vi "Dashboard Main.vi"() -> ()   [LabVIEW 2015]
uses:
  <vilib>/Utility/miscctls.llb/LVRowAndColumnTypeDef.ctl
  <vilib>/event_ctls.llb/eventvkey.ctl
  <vilib>/Rock Robotics/WPI/Dashboard/WPI_DashboardLogging Global.vi
  <vilib>/Rock Robotics/Network Tables/NT Read Boolean.vi
  <vilib>/Rock Robotics/Network Tables/NT Read Numeric Array.vi
  <vilib>/Utility/config.llb/Write Key (String).vi
  <vilib>/Utility/config.llb/Write Key (I32).vi
  <vilib>/Utility/config.llb/NI_LVConfig.lvlib
  <vilib>/vision/NI_Vision_Development_Module.lvlib
panel:
  out "Camera Image 2":T1(plugin-control)
  in  "Vision 2":u16(ring) items=["Camera Off", "USB Camera SW", "USB Camera HW", "IP Camera"]
  in  "Rec Mode":enum32{"Stop", "Record", "Playback"}(radio)
  in  "Vision":u16(ring) items=["Camera Off", "USB Camera SW", "USB Camera HW", "IP Camera"]
  in  "Dashboard Tab":T2(tab)
  out "Camera Reversed":bool
  out "dist":dbl
  in  "Select Auto":string(combo)
  out "NT Connection":bool
  in  "Camera Settings":T3={"Frame Rate"=30, "Compression"=30, "Size"=1} {"Frame Rate" scale=1.0..30.0; "Size" items=["640x480", "320x240", "160x120"]}
  out "MotorChart R":cluster{"Numeric":dbl, "Numeric":dbl}(graph)
  out "MotorChart L":T4(graph)
  out "MotorSliders R":cluster{"MotorSlide1":dbl, "MotorSlide2":dbl} {"MotorSlide2" scale=-1.0..1.0 scale format="%#_2e"; "MotorSlide1" scale=-1.0..1.0 scale format="%#_2e"}
  out "MotorSliders L":T5 {"MotorSlide4 2" scale=0.0..14.0 scale format="%#_2e"; "MotorSlide2" scale=-1.0..1.0 scale format="%#_2e"; "MotorSlide1" scale=-1.0..1.0 scale format="%#_2e"}
  out "Gyro":dbl(knob) scale=0.0..360.0
  out "JS1 Z":dbl(slide) scale=-1.0..1.0 scale format="%#_2e"
  out "JS1 Graph":cluster{"X":dbl, "Y":dbl}[](graph)
  out "JS1 Buttons":T6
  out "JS2 Z":dbl(slide) scale=-1.0..1.0 scale format="%#_2e"
  out "JS2 Graph":cluster{"X":dbl, "Y":dbl}[](graph)
  out "JS2 Buttons":T6
  out "Mode":T7(ring)=enum."Auto Disabled"
  in  "DB Camera Config":bool
  out "fps":dbl format="%#.1g"
  out "Mbps":dbl format="%#.1g"
  out "Mbps LED":bool
  in  "Camera Settings 2":T3={"Frame Rate"=30, "Compression"=30, "Size"=1} {"Frame Rate" scale=1.0..30.0; "Size" items=["640x480", "320x240", "160x120"]}
  out "Mbps 2":dbl format="%#.1g"
  out "fps 2":dbl format="%#.1g"
  out "Background":bool
  in  "DB/String 9":string
  in  "DB/String 8":string
  in  "DB/String 7":string
  in  "DB/String 6":string
  in  "DB/String 5":string
  in  "DB/String 4":string
  in  "DB/String 3":string
  in  "DB/String 2":string
  in  "DB/String 1":string
  in  "DB/String 0":string
  in  "DB/Slider 0":dbl(slide) scale=0.0..5.0
  in  "DB/Slider 1":dbl(slide) scale=0.0..5.0
  in  "DB/Slider 2":dbl(slide) scale=0.0..5.0
  in  "DB/Slider 3":dbl(slide) scale=0.0..5.0
  out "DB/LED 3":bool
  out "DB/LED 2":bool
  out "DB/LED 1":bool
  out "DB/LED 0":bool
  in  "DB/Button 3":bool
  in  "DB/Button 2":bool
  in  "DB/Button 1":bool
  in  "DB/Button 0":bool caption="New Name"
  in  "Test Slider":dbl(slide) scale=0.0..100.0 scale format="%#_3g"
  in  "On/Off":bool caption="Solenoid"
  in  "Test Name":u16(ring) items=["Select the test to run..."]
  in  "Test Tree":string(tree)
  in  "Motor":cluster{"Value":dbl, "Enable":bool} {"Value" scale=-1.0..1.0 scale format="%#_3g"}
  out "Progress":T8 {"Test Progress" scale=0.0..100.0}
  in  "Rev/Fwd":cluster{"Forward":bool, "Reverse":bool}
  in  "Test Ring":u16(ring) items=["Monochrome", "Color"]
  out "Cmd Status":string
  in  "Execute Command":bool
  in  "Command Params":string[][](table)
  in  "Command Selection":i32(listbox)
  in  "CheckList":i32(listbox)
  out "Tree":string(tree)
  in  "TCP":refnum<k5>
  out "Camera IP":string
  out "Image Message":string="Timeout in Camera Communications"
  out "Camera Image":T1(plugin-control)
  # "Left"
  # "Front"
  # "Right"
  # "Battery"
  # "This tab is a great place for autonomous settings and robot-specific values.\nPlace controls and indicators inside this tab and match name to\nDashboard Variables on robot. You can also delete this comment."
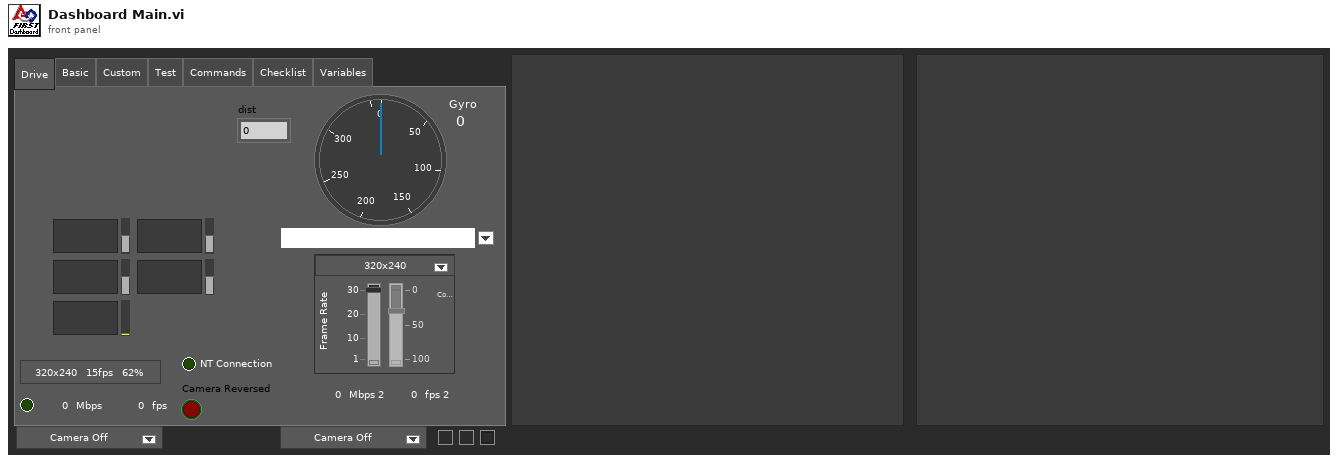
[diagram p1: front panel]
types:
  T1 = typedef "IMAQ Image.ctl" = refnum<image>
  T2 = enum32{"Drive", "Basic", "Custom", "Test", "Commands", "Checklist", "Variables"}
  T3 = cluster{"Frame Rate":i32, "Compression":i32, "Size":u16}
  T4 = cluster{"Numeric":dbl, "Numeric":dbl, "Battery V":dbl}
  T5 = cluster{"MotorSlide1":dbl, "MotorSlide2":dbl, "MotorSlide4 2":dbl}
  T6 = cluster{bool, bool, bool, bool, bool, bool, bool, bool, bool, bool, bool, bool}
  T7 = enum8{"Tele-Op Disabled", "Tele-Op Enabled", "Auto Disabled", "Auto Enabled", "Test Disabled", "Test Enabled", "Disconnected", "No Code", "E-Stop"}
  T8 = cluster{"Test Progress":u8, "Test Progress Text":string}
  T9 = typedef "Image Type" = u32
  T10 = cluster{"IDs":cluster{"RPC field ID":u16, "Unique ID":u16}, "String":string}
  T11 = enum32{"Drive", "Basic", "Custom", "Test", "Checklist", "Variables"}
  T12 = cluster{"Camera Image":refnum<vi>, "Dashboard Tab":refnum<vi>, "Background":refnum<vi>, "Vision":refnum<vi>, "Rec Mode":refnum<vi>, "Test Slider":refnum<vi>, "On/Off ":refnum<vi>, "Test Ring":refnum<vi>, "Rev/Fwd":refnum<vi>, "Test Name":refnum<vi>, "Motor":refnum<vi>, "Progress":refnum<vi>, "CheckList":refnum<vi>, "Tree":refnum<vi>, "Test Tree":refnum<vi>, "Command Params":refnum<vi>, "Command Selection":refnum<vi>, "Execute Command":refnum<vi>, "Cmd Status":refnum<vi>}
  T13 = cluster{"Error Strings":string, "Disable Counts":cluster{u16, u16}, "Rail Faults":cluster{u16, u16, u16}, "Robot IP":string, "DB Mode":u8, "Event Info":cluster{"Name":string, "Type":u8, "Number":u16, "Replay":u8}, "Camera Addr":string}
  T14 = cluster{"Storage":cluster{"Disk Free":u64, "RAM Block":u32, "RAM free":u32}, "CPU Utilization":cluster{"CPU % ISR":sgl, "CPU % Time Crit":sgl, "CPU % Timed Str":sgl, "CPU % High":sgl, "CPU % Above":sgl, "CPU % Normal":sgl, "CPU % Low":sgl}, "CAN":cluster{"% Bus Utilization":sgl, "Bus Off Cnt":u32, "TX_FIFO Full Cnt":u32, "Receive Error Cnt":u8, "Transmit Error Cnt":u8}, "HID":cluster{"HID Outputs":u32, "Rumble Low":u16, "Rumble High":u16}[]}
  T15 = cluster{"Status bits":cluster{"Test Mode":bool, "Autonomous":bool, "Enabled":bool, "Code Start":bool, "Brownout":bool, "Reserved 2":bool, "Reserved 3":bool, "E-Stop":bool}, "Code Trace":cluster{"Disabled":bool, "TeleOp":bool, "Auto":bool, "Test":bool}, "Controller Type":enum16{"unknown", "cRIO", "roboRio"}, "Code?":enum16{"unknown", "noCode", "code"}, "Battery V":dbl}
  T16 = cluster{"Control Bits":cluster{"TestMode":bool, "Autonomous":bool, "Enabled":bool, "FMS Present":bool, bool, bool, bool, "E-Stop":bool}, "Team Station ":u8, "Countdown":sgl, "Joystick Values":cluster{"Axes":dbl[], "Buttons":bool[], "POVs":i16[]}[]}
  T17 = cluster{"Axes":dbl[], "Buttons":bool[], "POVs":i16[]}[]
  T18 = cluster{"Axes":dbl[], "Buttons":bool[], "POVs":i16[]}
  T19 = cluster{"Buttons[0]":bool, "Buttons[1]":bool, "Buttons[2]":bool, "Buttons[3]":bool, "Buttons[4]":bool, "Buttons[5]":bool, "Buttons[6]":bool, "Buttons[7]":bool, "Buttons[8]":bool, "Buttons[9]":bool, "Buttons[10]":bool, "Buttons[11]":bool}
  T20 = typedef "NI_LVConfig.lvlib/Config Data RefNum.ctl" = refnum<k1>
  T21 = cluster{"Operation":enum16{"Update", "Clear"}, "Color Box":u32}[]
  T22 = typedef "eventvkey.ctl" = enum16{"ASCII", "Enter", "Return", "Shift", "Ctrl", "Alt", "Cmd", "Opt", "Caps", "NumLock", "Clear", "Break", "Up", "Down", "Left", "Right", "Insert", "Delete", "Home", "End", "PageUp", "PageDown", "Escape", "Help", "Pause", "ScrollLock", "F1", "F2", "F3", "F4", "F5", "F6", "F7", "F8", "F9", "F10", "F11", "F12", "F13", "F14", "F15", "F16", "F17", "F18", "F19", "F20", "F21", "F22", "F23", "F24", "Play", "VolumeUp", "VolumeDown", "Mute", "Two Byte Char"}
  T23 = cluster{"Image Size":bool, "Image Type":bool, "Pixel Value":bool, "ROI Information":bool, "Zoom Factor":bool}
  T24 = enum8{"Enabled", "Disabled", "Disabled and Grayed Out"}
  T25 = cluster{"Operation":enum16{"Update", "Clear"}, "Color Box":u32}
  T26 = typedef "LVRowAndColumnTypeDef.ctl" = cluster{"Row":i32, "Column":i32}
  T27 = cluster{"Shift":bool, "Ctrl":bool, "Alt":bool, "Cmd":bool, "Opt":bool}
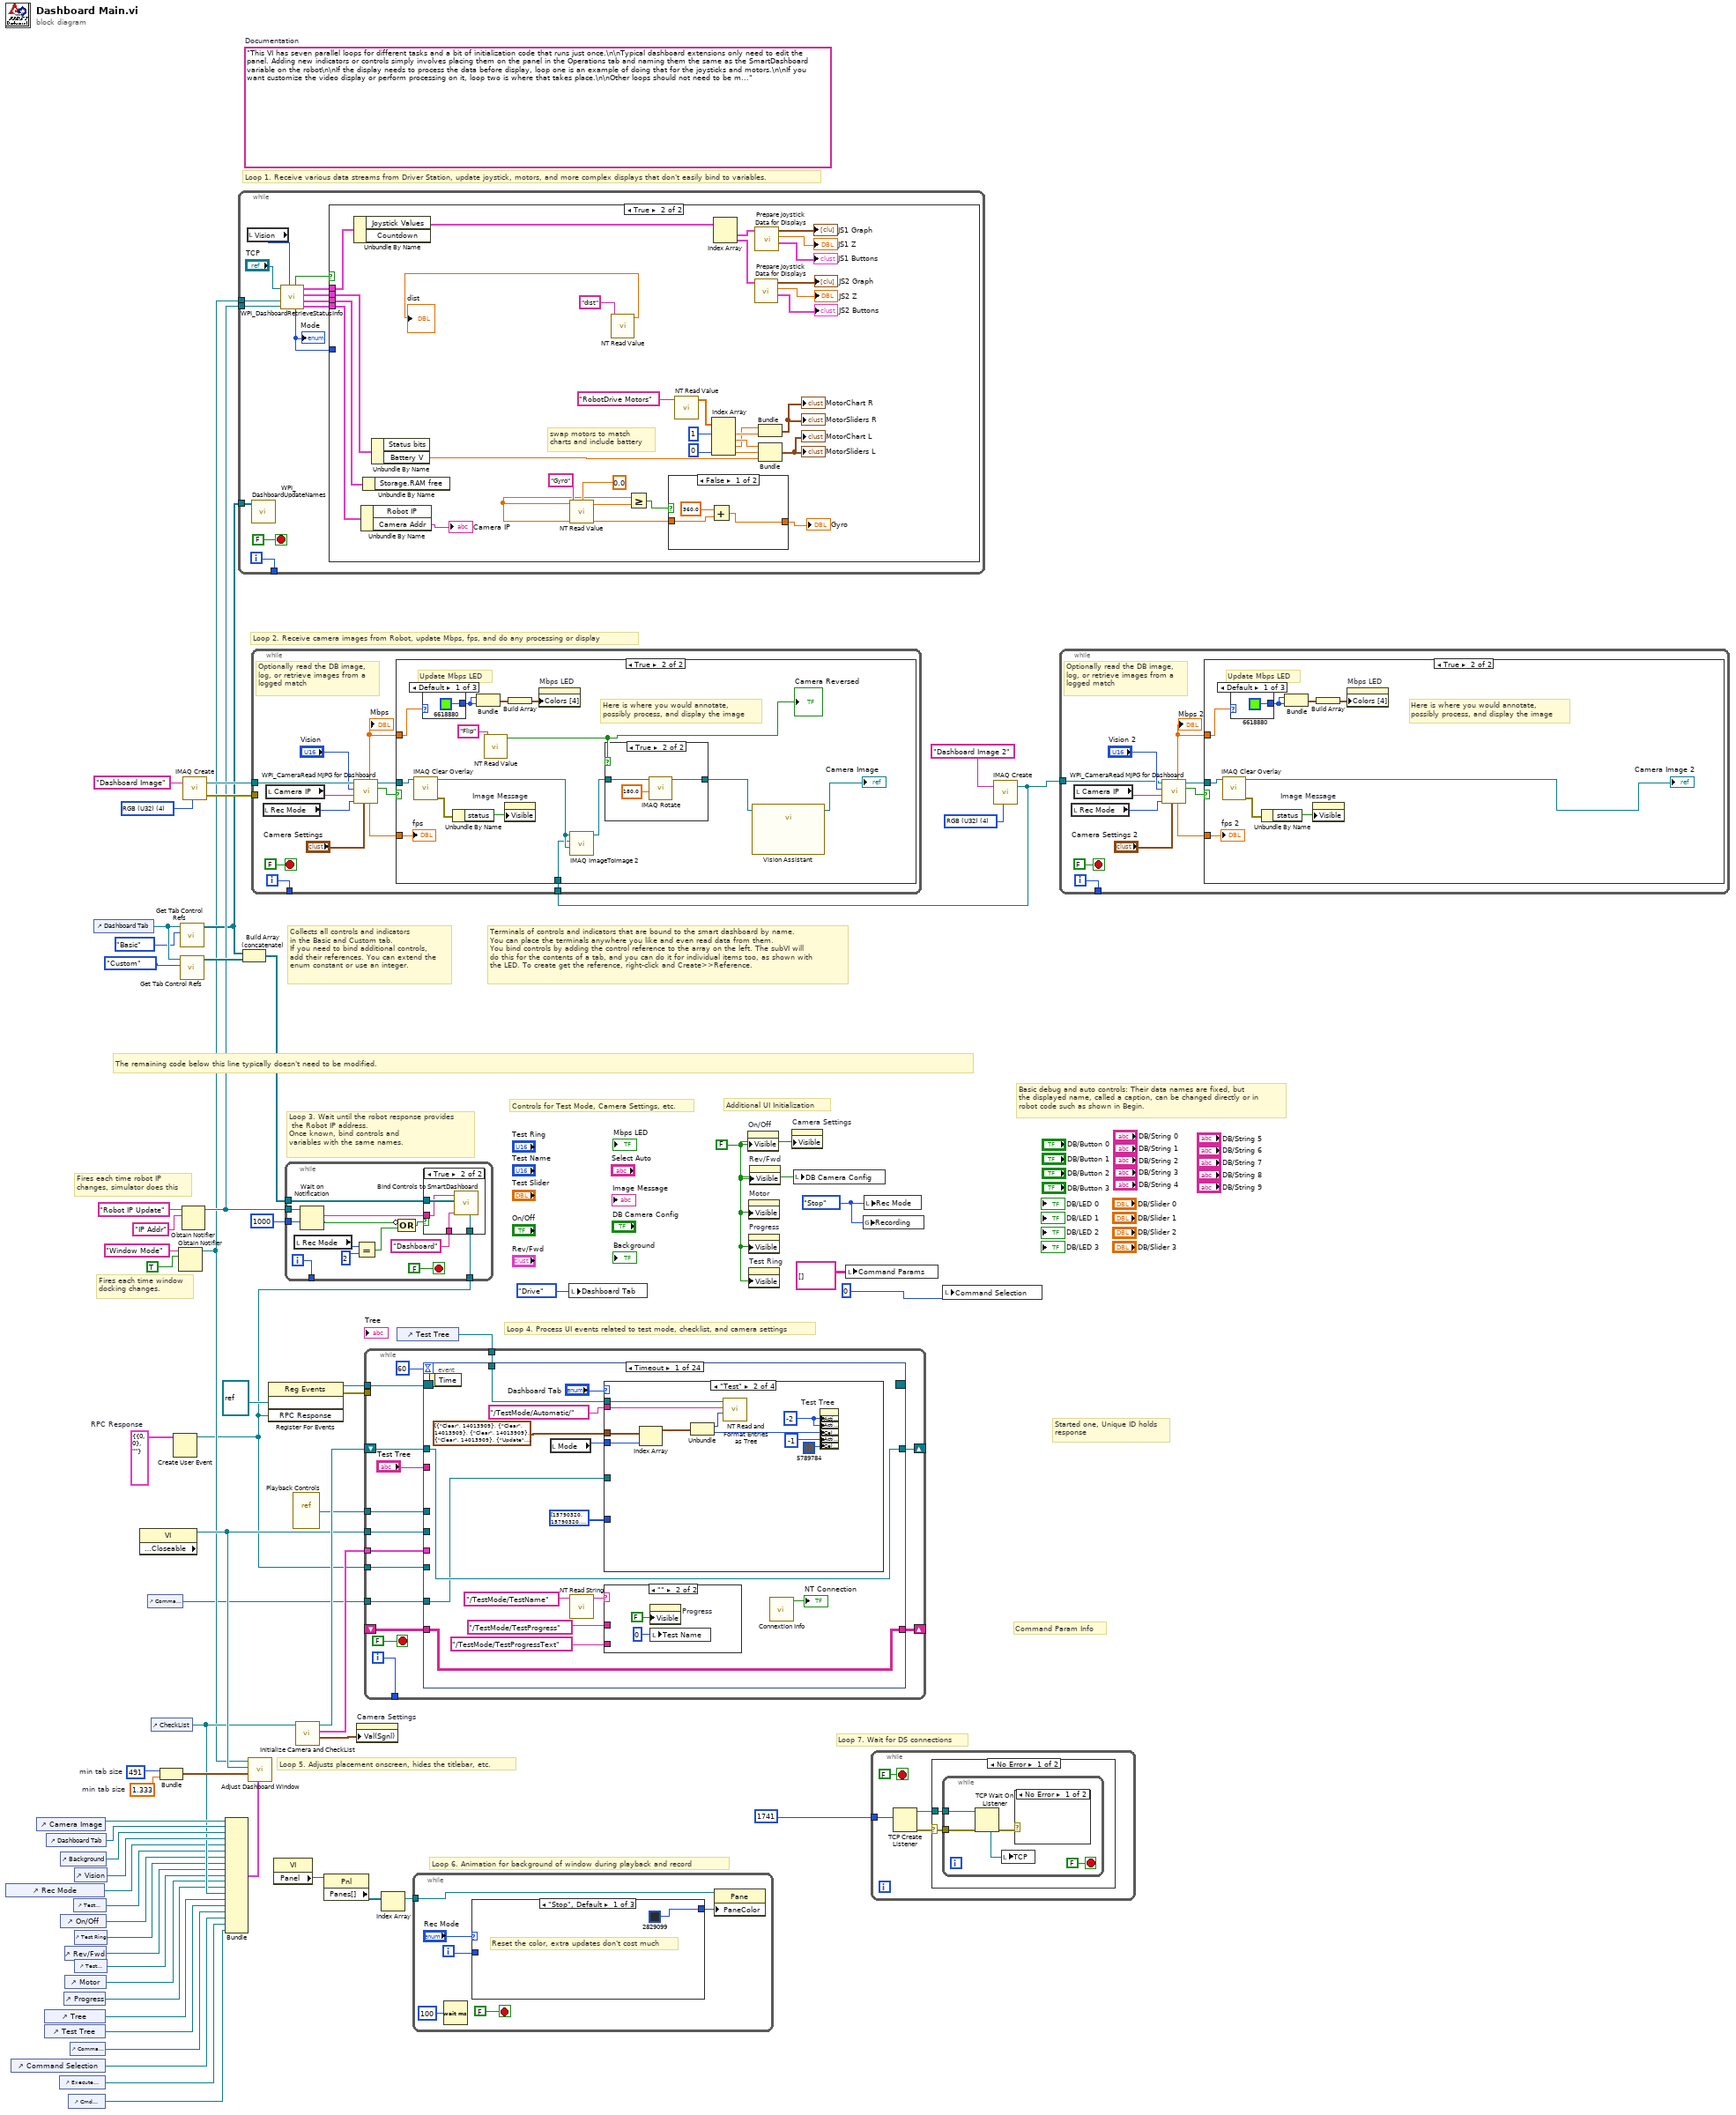
[diagram p0: block diagram]
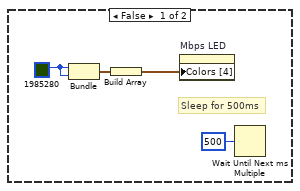
[diagram p2: hidden frame]
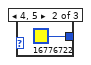
[diagram p3: hidden frame]
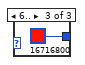
[diagram p4: hidden frame]
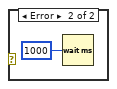
[diagram p5: hidden frame]
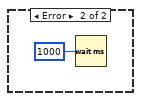
[diagram p6: hidden frame]
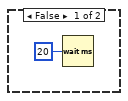
[diagram p7: hidden frame]
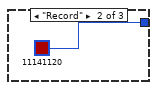
[diagram p9: hidden frame]
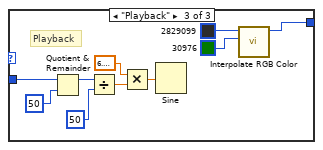
[diagram p10: hidden frame]
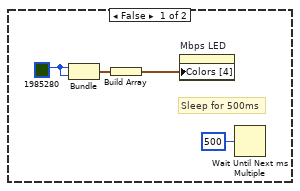
[diagram p12: hidden frame]
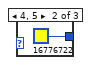
[diagram p14: hidden frame]
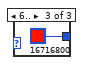
[diagram p15: hidden frame]
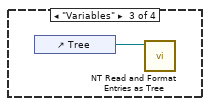
[diagram p17: hidden frame]
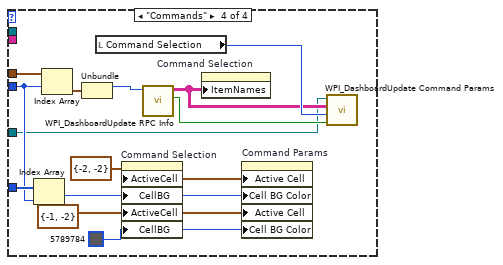
[diagram p18: hidden frame]
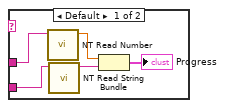
[diagram p19: hidden frame]
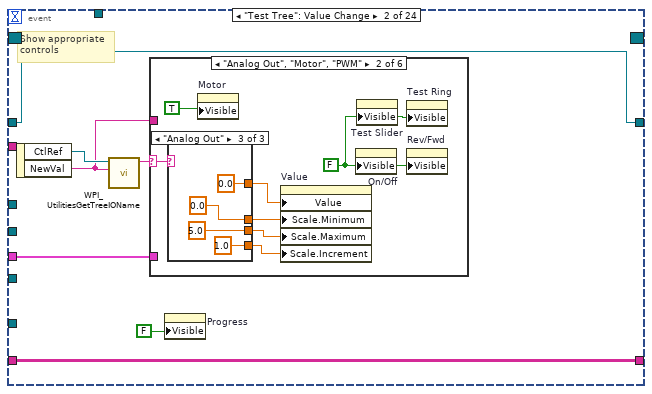
[diagram p20: hidden frame]
diagram:
  w2 = T9 4 items=["Grayscale (U8)", "Grayscale (I16)", "Grayscale (SGL)", "Complex (CSG)", "RGB (U32)", "HSL (U32)", "RGB (U64)", "Grayscale (U16)"] ("Image Type")
  w10 = T10 {"IDs"={"RPC field ID"=0, "Unique ID"=0}, "String"=""}  # RPC Response
  w36 = 491  # min tab size
  w35 = 1.333  # min tab size
  w44 = enum32{"Stop", "Record", "Playback"}."Stop" ("Rec Mode")
  w18 = FALSE ("Visible")
  (unwired) "This VI has seven parallel loops for different tasks and a bit of initialization code that runs just once.\n\nTypical dashboard extensions only need to edit the panel. Adding new indicators or controls simply involves placing them on the panel in the Operations tab and naming them the same as the SmartDashboard variable on the robot\n\nIf the display needs to process the data before display, loop one is an example of doing that for the joysticks and motors.\n\nIf you want customize the video display or perform processing on it, loop two is where that takes place.\n\nOther loops should not need to be modified. They are pretty standard, and document the task they perform."  # Documentation
  w64 = T9 4 items=["Grayscale (U8)", "Grayscale (I16)", "Grayscale (SGL)", "Complex (CSG)", "RGB (U32)", "HSL (U32)", "RGB (U64)"] ("Image Type")
  # "Command Param Info"
  # "Started one, Unique ID holds\nresponse"
  # "Loop 7. Wait for DS connections"
  # "Basic debug and auto controls: Their data names are fixed, but\nthe displayed name, called a caption, can be changed directly or in\nrobot code such as shown in Begin."
  # "Controls for Test Mode, Camera Settings, etc."
  # "Additional UI Initialization"
  # "Loop 6. Animation for background of window during playback and record"
  # "Fires each time robot IP\nchanges, simulator does this"
  # "Fires each time window\ndocking changes."
  # "Collects all controls and indicators\nin the Basic and Custom tab.\nIf you need to bind additional controls,\nadd their references. You can extend the\nenum constant or use an integer."
  # "The remaining code below this line typically doesn't need to be modified."
  # "Loop 4. Process UI events related to test mode, checklist, and camera settings"
  # "Terminals of controls and indicators that are bound to the smart dashboard by name.\nYou can place the terminals anywhere you like and even read data from them.\nYou bind controls by adding the control reference to the array on the left. The subVI will\ndo this for the contents of a tab, and you can do it for individual items too, as shown with\nthe LED. To create get the reference, right-click and Create>>Reference."
  # "Loop 3. Wait until the robot response provides\n the Robot IP address.\nOnce known, bind controls and\nvariables with the same names."
  # "Loop 5. Adjusts placement onscreen, hides the titlebar, etc."
  # "Loop 1. Receive various data streams from Driver Station, update joystick, motors, and more complex displays that don't easily bind to variables."
  # "Loop 2. Receive camera images from Robot, update Mbps, fps, and do any processing or display"
  n1 = control-ref of="Rec Mode"() -> (w24:refnum<vi>)
  n2 = control-ref of="Command Selection"() -> (w9:refnum<vi>)
  n3 = control-ref of="Camera Image"() -> (w39:refnum<vi>)
  n4 = control-ref of="Tree"() -> (w28:refnum<vi>)
  n5 = control-ref of="Test Tree"() -> (w27:refnum<vi>)
  n6 = control-ref of="Dashboard Tab"() -> (w38:refnum<vi>)
  n7 = control-ref of="Execute Command"() -> (w11:refnum<vi>)
  n8 = control-ref of="Background"() -> (w33:refnum<vi>)
  n9 = control-ref of="On/Off"() -> (w22:refnum<vi>)
  n10 = control-ref of="Progress"() -> (w19:refnum<vi>)
  n11 = control-ref of="Rev/Fwd"() -> (w20:refnum<vi>)
  n12 = control-ref of="Motor"() -> (w25:refnum<vi>)
  n13 = control-ref of="Cmd Status"() -> (w5:refnum<vi>)
  n14 = control-ref of="Command Params"() -> (w12:refnum<vi>)
  n15 = control-ref of="Test Slider"() -> (w23:refnum<vi>)
  n16 = control-ref of="Vision"() -> (w37:refnum<vi>)
  n17 = control-ref of="Test Ring"() -> (w21:refnum<vi>)
  n18 = control-ref of="Test Name"() -> (w26:refnum<vi>)
  n19 = control-ref of="Dashboard Tab"() -> (w42:refnum<vi>)
  n20 = property class="VI" props=["Front Panel.Closeable"]() -> (reference out=w43:refnum<vi>)  [unwired: 2 in, 2 out]
  n21 = control-ref of="Command Params"() -> (w4:refnum<vi>)
  n22 = control-ref of="CheckList"() -> (w29:refnum<vi>)
  n23 = Bundle("min tab size"=w36, "min tab size"=w35) -> (w34:cluster{"min tab size":i32, "min tab size":dbl})  [unwired: 1 in]
  n24 = Create User Event(user event datatype=w10) -> (user event=w6:refnum<user-event>)  [unwired: 1 in, 1 out]
  n25 = Obtain Notifier(name (unnamed)="Window Mode", notification data type=TRUE) -> (notifier out=w15:refnum<notifier>)  [unwired: 2 in, 2 out]
  n26 = call <vilib>:"Get Tab Control Refs.vi"("Page Index"=T11."Basic" ("Dashboard Tab"), "TabControl in"=w42) -> ("ControlsOnPage"=w16:refnum<vi>[])  [unwired: 9 in]
  n27 = call <vilib>:"Get Tab Control Refs.vi"("Page Index"=T11."Custom" ("Dashboard Tab"), "TabControl in"=w42) -> ("ControlsOnPage"=w41:refnum<vi>[])  [unwired: 9 in]
  n28 = Obtain Notifier(name (unnamed)="Robot IP Update", notification data type="IP Addr" ("name (unnamed)")) -> (notifier out=w17:refnum<notifier>)  [unwired: 2 in, 2 out]
  n29 = call "IMAQ Create"("Image Name"="Dashboard Image", "Image Type"=w64) -> ("New Image"=w62:T1, "error out"=w61:errorcluster)  [unwired: 2 in, 1 out]
  n30 = Bundle("Camera Image"=w39, "Dashboard Tab"=w38, "Background"=w33, "Vision"=w37, "Rec Mode"=w24, "Test Slider"=w23, "On/Off"=w22, "Test Ring"=w21, "Rev/Fwd"=w20, "Test Name"=w26, "Motor"=w25, "Progress"=w19, "CheckList"=w29, "Tree"=w28, "Test Tree"=w27, "Command Params"=w12, "Command Selection"=w9, "Execute Command"=w11, "Cmd Status"=w5) -> (w30:T12)  [unwired: 1 in]
  n31 = while {
    tunnel: [w76] -> _
    tunnel: w17 -> [w70]
    tunnel: w16 -> [w69]
    tunnel: w15 -> [w65]
    i -> [w76]
    stop <- FALSE stop-if-true
    n32 = local read "Vision"() -> (w67:u16)
    n33 = call <vilib>:"WPI_DashboardUpdateNames.vi"("Controls on Tab"=w69) -> ()  [unwired: 11 in]
    n34 = call <vilib>:"WPI_DashboardRetrieveStatusInfo.vi"("Vision"=w67, "Binding Refnum"=w70, "Window Mode Notifier"=w65, "TCP Cnx"="TCP") -> ("Power and Errors"=w71:T13, "Robot Metrics"=w74:T14, "Status Info"=w75:T15, "Control Info"=w72:T16, "Robot Mode"=w68:T7, "Process?"=w73:bool)  [unwired: 2 in]
    "Mode" <- w68
    n35 = case shown="True" w73 {
      tunnel: w75 -> [_ w110]
      tunnel: w74 -> [_ w109]
      tunnel: w72 -> [_ w108]
      tunnel: w71 -> [_ w107]
      tunnel: w68 -> [_ _]
      frame False {
        n36 = Wait (ms)(milliseconds to wait=u32 20) -> ()  [unwired: 1 out]
      }
      frame True {
        # "swap motors to match\ncharts and include battery"
        n37 = Unbundle By Name(w108) -> ("Joystick Values"=w97:T17)  [unwired: 1 out]
        n38 = Unbundle By Name(w107) -> ("Camera Addr"=→"Camera IP":string)  [unwired: 1 out]
        n39 = Unbundle By Name(w109) -> ()  [unwired: 1 out]
        n40 = Unbundle By Name(w110) -> ("Battery V"=w98:dbl)  [unwired: 1 out]
        n41 = call-poly <vilib>:"NT Read Value.vi"("Name"="Gyro") -> ("Numeric"=w82:dbl)  [unwired: 9 in, 1 out]
        n42 = call-poly <vilib>:"NT Read Value.vi"("Name"="dist") -> ("Numeric"=→"dist":dbl)  [unwired: 9 in, 1 out]
        n43 = Greater Or Equal?(x=w82, y=0.0) -> (x >= y?=w84:bool)
        n44 = case shown="False" w84 {
          tunnel: [w111 w114] -> w81
          tunnel: w82 -> [w112 w114]
          frame False {
            n45 = Add(x=360.0, y=w112) -> (x+y=w111:dbl)
          }
          frame True {
          }
        }
        "Gyro" <- w81
        n46 = call-poly <vilib>:"NT Read Value.vi"("Name"="RobotDrive Motors") -> ("Numeric Array"=w86:dbl[])  [unwired: 9 in, 1 out]
        n47 = Index Array(array=w86, index #1=1, index #4=0) -> (element #1=w102:dbl, element #2=w103:dbl, element #3=w101:dbl, element #4=w106:dbl)  [unwired: 2 in]
        n48 = Index Array(array=w97) -> (element #1=w96:T18, element #2=w91:T18)  [unwired: 2 in]
        n49 = call "Prepare Joystick Data for Displays.vi"("Joystick Values"=w91) -> ("Buttons"=→"JS2 Buttons":T19, "Z Axis"=→"JS2 Z":dbl, "Cartesian Data"=→"JS2 Graph":cluster{"X axis":dbl, "X axis":dbl}[])  [unwired: 8 in]
        n50 = call "Prepare Joystick Data for Displays.vi"("Joystick Values"=w96) -> ("Buttons"=→"JS1 Buttons":T19, "Z Axis"=→"JS1 Z":dbl, "Cartesian Data"=→"JS1 Graph":cluster{"X axis":dbl, "X axis":dbl}[])  [unwired: 8 in]
        n51 = Bundle("Numeric"=w101, "Numeric"=w102) -> (→"MotorChart R" →"MotorSliders R":cluster{"Numeric":dbl, "Numeric":dbl})  [unwired: 1 in]
        n52 = Bundle("Numeric"=w103, "Numeric"=w106, "Battery V"=w98) -> (→"MotorChart L" →"MotorSliders L":T4)  [unwired: 1 in]
      }
    }
  }
  n53 = Build Array (concatenate)(w16, w41) -> (w40:refnum<vi>[])
  n54 = call "Adjust Dashboard Window.vi"("Sizing Refnums"=w30, "Size Constraints"=w34, "VI"=w43, "WIn Mode"=w15) -> ()  [unwired: 8 in]
  n55 = register-events(refnum<vi> refnum, w6) -> (reference out=w48:refnum<event-registration>, error out=w47:errorcluster)  [unwired: 2 in]
  n56 = property class="VI"() -> ("Panel"=w51:refnum<vi>)  [unwired: 2 in, 2 out]
  n57 = while {
    tunnel: w40 -> [w127]
    tunnel: w17 -> [w125]
    tunnel: [w123] -> _
    tunnel: u32 1000 ("milliseconds to wait") -> [w122]
    tunnel: w6 -> [w115]
    i -> [w123]
    stop <- FALSE stop-if-true
    n58 = local read "Rec Mode"() -> (w118:enum32{"Stop", "Record", "Playback"})
    n59 = Wait on Notification(notifier=w125, timeout in ms (-1)=w122) -> (notification=w124:string, timed out?=w120:bool)  [unwired: 2 in, 2 out]
    n60 = Equal?(x=w118, y=u16 2 ("Rec Mode")) -> (x = y?=w119:bool)
    n61 = Compound Arithmetic op=OR(invert w120, w119) -> (w121:bool)
    n62 = case shown="True" w121 {
      tunnel: w127 -> [_ w131]
      tunnel: w124 -> [_ w130]
      tunnel: "Dashboard" -> [_ w129]
      tunnel: w115 -> [_ w128]
      frame False {
      }
      frame True {
        n63 = call <vilib>:"Bind Controls to SmartDashboard.vi"("RPC ref"=w128, "Client Name"=w129, "Bound Control Refs"=w131, "Server IP Address"=w130) -> ()  [unwired: 8 in]
      }
    }
  }
  n64 = vi-ref "Playback Controls.vi"() -> (w49:refnum<vi>)
  n65 = call "Initialize Camera and CheckList.vi"("ListBox in"=w29) -> ("Cluster"=w55:cluster{"value":i32, "value":i32, "index":i32}, "Array"=w56:cluster{string[]}[], "File Refnum"=w54:T20)  [unwired: 8 in]
  n66 = property class="Pnl"(reference=w51) -> ("Panes[]"=w52:refnum<vi>[])  [unwired: 1 in, 2 out]
  n67 = property on="Camera Settings" class="Clust (strict)"("Val(Sgnl)"=w55) -> ()  [unwired: 2 in, 2 out]
  n68 = Index Array(array=w52) -> (element=w50:refnum<vi>)  [unwired: 1 in]
  n69 = control-ref of="Test Tree"() -> (w53:refnum<vi>)
  n70 = while {
    tunnel: w56 -> [w143]
    shift-right: [w142] -> _
    shift-left: w54 -> [w141]
    tunnel: [w140] -> _
    tunnel: w53 -> [w139]
    tunnel: w49 -> [w138]
    tunnel: w48 -> [w137]
    tunnel: w47 -> [_]
    tunnel: w43 -> [w136]
    tunnel: w6 -> [w135]
    tunnel: w4 -> [w134]
    shift-right: [w133] -> _
    shift-left: _ -> [w132]
    i -> [w140]
    stop <- FALSE stop-if-true
    n71 = event shown="[0] Timeout" {
      selector: w137 -> [_ _ _ _ _ _ _ _ _ _ _ _ _ _ _ _ _ _ _ _ _ _ _ _]
      dyn-events: [_ _ _ _ _ _ _ _ _ _ _ _ _ _ _ _ _ _ w452 _ _ _ _ _] -> _
      timeout: u32 60 ("milliseconds to wait") -> [_ _ _ _ _ _ _ _ _ _ _ _ _ _ _ _ _ _ _ _ _ _ _ _]
      tunnel: w139 -> [w156 _ _ _ _ _ _ _ _ _ _ _ _ _ _ _ _ _ _ _ _ _ _ _]
      tunnel: "Test Tree" -> [_ _ _ _ _ _ _ _ _ _ _ _ _ w415 w424 w427 w432 w441 _ _ _ _ _ _]
      tunnel: w143 -> [_ w194 _ _ _ _ _ _ _ _ _ w377 w408 _ _ _ _ _ _ _ _ _ _ _]
      tunnel: [w153 w193 w297 w303 w313 w317 w323 w335 w343 w349 w362 w376 w401 w414 w422 w426 w431 w440 w454 w470 w472 w480 w491 w496] -> w142
      tunnel: w141 -> [w153 w193 w297 w303 w313 w317 w323 w335 w343 w349 w362 w375 w401 w414 w422 w426 w431 w440 w454 w470 w472 w480 w491 w496]
      tunnel: w138 -> [_ _ _ _ _ _ _ _ _ _ _ _ _ _ _ _ _ _ w455 _ w475 _ _ _]
      tunnel: w136 -> [_ _ _ _ _ _ _ _ _ _ _ _ _ _ _ _ _ _ w450 _ _ _ _ _]
      tunnel: w135 -> [_ _ _ _ _ _ _ _ _ _ _ _ _ _ _ _ _ _ w446 _ _ _ _ _]
      tunnel: w134 -> [w148 _ _ _ _ _ w321 _ _ _ _ _ _ _ _ _ _ _ _ _ _ _ _ _]
      tunnel: [w147 w192 w296 w302 w312 w318 w319 w329 w340 w348 w361 w374 w400 w413 w421 w425 w430 w439 w445 w468 w471 w476 w484 w497] -> w133
      tunnel: w132 -> [w147 w192 w296 w302 w312 w318 w319 _ _ w348 w361 w374 w400 w413 w421 w425 w430 w439 w445 w468 w471 w476 w484 w497]
      event Timeout {
        n72 = event-data() -> ()  [unwired: 1 in, 1 out]
        n73 = local read "Mode"() -> (w150:T7)
        n74 = call <vilib>:"NT Read String.vi"("Name"="/TestMode/TestName") -> ("String"=w159:string)  [unwired: 9 in, 1 out]
        n75 = case shown="\"Test\"" "Dashboard Tab" {
          tunnel: w156 -> [_ w170 _ _]
          tunnel: "/TestMode/Automatic/" ("Name Pattern") -> [_ w169 _ _]
          tunnel: T21 [{"Operation"=enum."Clear", "Color Box"=14013909}, {"Operation"=enum."Clear", "Color Box"=14013909}, {"Operation"=enum."Clear", "Color Box"=14013909}, {"Operation"=enum."Clear", "Color Box"=14013909}, {"Operation"=enum."Update", "Color Box"=14013909}, {"Operation"=enum."Update", "Color Box"=16777215}, {"Operation"=enum."Clear", "Color Box"=14013909}, {"Operation"=enum."Clear", "Color Box"=14013909}, {"Operation"=enum."Clear", "Color Box"=14013909}] -> [_ w162 _ w179]
          tunnel: w150 -> [_ w161 _ w178]
          tunnel: u32[] [15790320, 15790320, 15790320, 15790320, 16777215, 16777215, 15790320, 15790320, 15790320] -> [_ _ _ w184]
          tunnel: w148 -> [_ _ _ w172]
          frame "Custom", Default {
          }
          frame "Test" {
            w168 = -2 ("Active Item:Row Number")
            n76 = Index Array(array=w162, index=w161) -> (element=w163:T25)
            n77 = Unbundle(w163) -> ("Operation"=w164:enum16{"Update", "Clear"}, "Color Box"=w165:u32)
            n78 = call <vilib>:"NT Read and Format Entries as Tree.vi"("Operation"=w164, "Name Pattern"=w169, "Tree Refnum"=w170) -> ()  [unwired: 7 in, 2 out]
            n79 = property on="Test Tree" class="Tree (strict)"("Active Item Row Number"=w168, "ActiveColNum"=w168, "CellBG"=w165, "Active Item Row Number"=-1 ("Active Item:Row Number"), "CellBG"=u32 5789784 ("Color Box")) -> ()  [unwired: 2 in, 2 out]
          }
          frame "Variables" {
            n80 = control-ref of="Tree"() -> (w171:refnum<vi>)
            n81 = call <vilib>:"NT Read and Format Entries as Tree.vi"("Tree Refnum"=w171) -> ()  [unwired: 9 in, 2 out]
          }
          frame "Commands" {
            w180 = u32 5789784 ("Color Box")
            w181 = T26 {"Row"=-1, "Column"=-2} ("Active Cell:Active Cell")
            w183 = T26 {"Row"=-2, "Column"=-2} ("Active Cell:Active Cell")
            n82 = Index Array(array=w184, index=w178) -> (element=w182:u32)
            n83 = Index Array(array=w179, index=w178) -> (element=w177:T25)
            n84 = Unbundle(w177) -> ("Operation"=w176:enum16{"Update", "Clear"})  [unwired: 1 out]
            n85 = local read "Command Selection"() -> (w175:i32)
            n86 = property on="Command Selection" class="MCListbox (strict)"("ActiveCell"=w183, "CellBG"=w182, "ActiveCell"=w181, "CellBG"=w180) -> ()  [unwired: 2 in, 2 out]
            n87 = call <vilib>:"WPI_DashboardUpdate RPC Info.vi"("Operation"=w176) -> ("update"=w174:bool, "commands"=w173:string[][])  [unwired: 9 in]
            n88 = property on="Command Selection" class="MCListbox (strict)"("ItemNames"=w173) -> ()  [unwired: 2 in, 2 out]
            n89 = property on="Command Params" class="Tbl (strict)"("Active Cell"=w183, "Cell BG Color"=w182, "Active Cell"=w181, "Cell BG Color"=w180) -> ()  [unwired: 2 in, 2 out]
            n90 = call <vilib>:"WPI_DashboardUpdate Command Params.vi"("Update"=w174, "NewVal"=w175, "Commands"=w173, "Param Tbl"=w172) -> ()  [unwired: 7 in, 1 out]
          }
        }
        n91 = case shown="\"\"" w159 {
          tunnel: "/TestMode/TestProgress" ("Name") -> [w186 _]
          tunnel: "/TestMode/TestProgressText" ("Name") -> [w185 _]
          frame Default {
            n92 = call <vilib>:"NT Read Number.vi"("Name"=w186) -> ("Numeric"=w187:dbl)  [unwired: 9 in, 1 out]
            n93 = call <vilib>:"NT Read String.vi"("Name"=w185) -> ("String"=w188:string)  [unwired: 9 in, 1 out]
            n94 = Bundle("Numeric"=w187, "String"=w188) -> (→"Progress":cluster{"Numeric":dbl, "String":string})  [unwired: 1 in]
          }
          frame "" {
            n95 = property on="Progress" class="Clust (strict)"("Visible"=FALSE) -> ()  [unwired: 2 in, 2 out]
            n96 = local write "Test Name"(u16 0) -> ()
          }
        }
        n97 = call <vilib>:"Connextion Info.vi"() -> ("Connected"=→"NT Connection":bool)  [unwired: 10 in, 1 out]
      }
      event "Test Tree": Value Change {
        # "Show appropriate\ncontrols"
        n98 = event-data() -> ("CtlRef"=w197:refnum<vi>, "NewVal"=w195:string)  [unwired: 1 in]
        n99 = call <vilib>:"WPI_UtilitiesGetTreeIOName.vi"("NewVal"=w195, "TreeControl in"=w197) -> ("I/O Name"=w198:string)  [unwired: 9 in]
        n100 = case shown="\"Analog Out\", \"Motor\", \"PWM\"" w198 {
          selector: w198 -> [_ w205 _ w227 w236 _]
          tunnel: w195 -> [_ _ w224 w226 _ w243]
          tunnel: w194 -> [_ _ _ _ _ w242]
          frame Default {
            w200 = FALSE ("Visible")
            w199 = FALSE ("Visible")
            n101 = property on="Motor" class="Clust (strict)"("Visible"=w199) -> ()  [unwired: 2 in, 2 out]
            n102 = property on="Test Ring" class="Ring (strict)"("Visible"=w199) -> ()  [unwired: 2 in, 2 out]
            n103 = property on="Rev/Fwd" class="Clust (strict)"("Visible"=w200) -> ()  [unwired: 2 in, 2 out]
            n104 = property on="On/Off" class="Bool (strict)"("Visible"=w200) -> ()  [unwired: 2 in, 2 out]
            n105 = property on="Test Slider" class="Slide (strict)"("Visible"=w200) -> ()  [unwired: 2 in, 2 out]
          }
          frame "Analog Out", "Motor", "PWM" {
            w206 = FALSE ("Visible")
            n106 = case shown="\"Analog Out\"" w205 {
              tunnel: [1.0 ("Value") -1.0 ("Value") 0.0 ("Value")] -> w204
              tunnel: [255.0 ("Value") 1.0 ("Value") 5.0 ("Value")] -> w203
              tunnel: [128.0 ("Value") 0.0 ("Value") 0.0 ("Value")] -> w202
              tunnel: [64.0 ("Value") 0.5 ("Value") 1.0 ("Value")] -> w201
              frame "PWM" {
              }
              frame "Motor", Default {
              }
              frame "Analog Out" {
              }
            }
            n107 = property on="Motor" class="Clust (strict)"("Visible"=TRUE) -> ()  [unwired: 2 in, 2 out]
            n108 = property on="Value" class="Slide (strict)"("Value"=w202, "Scale.Minimum"=w204, "Scale.Maximum"=w203, "Scale.Increment"=w201) -> ()  [unwired: 2 in, 2 out]
            n109 = property on="On/Off" class="Bool (strict)"("Visible"=w206) -> ()  [unwired: 2 in, 2 out]
            n110 = property on="Test Slider" class="Slide (strict)"("Visible"=w206) -> ()  [unwired: 2 in, 2 out]
            n111 = property on="Test Ring" class="Ring (strict)"("Visible"=w206) -> ()  [unwired: 2 in, 2 out]
            n112 = property on="Rev/Fwd" class="Clust (strict)"("Visible"=w206) -> ()  [unwired: 2 in, 2 out]
          }
          frame "Servo" {
            w222 = FALSE ("Visible")
            n113 = call <vilib>:"NT Read Number.vi"("Name"=w224) -> ("Numeric"=w223:dbl)  [unwired: 9 in, 1 out]
            n114 = property on="Test Slider" class="Slide (strict)"("Visible"=TRUE, "Scale.Maximum"=170.0 ("Scale.Range:Maximum")) -> ()  [unwired: 2 in, 2 out]
            n115 = local write "Test Slider"(w223) -> ()
            n116 = property on="Motor" class="Clust (strict)"("Visible"=w222) -> ()  [unwired: 2 in, 2 out]
            n117 = property on="Rev/Fwd" class="Clust (strict)"("Visible"=w222) -> ()  [unwired: 2 in, 2 out]
            n118 = property on="On/Off" class="Bool (strict)"("Visible"=w222) -> ()  [unwired: 2 in, 2 out]
            n119 = property on="Test Ring" class="Ring (strict)"("Visible"=w222) -> ()  [unwired: 2 in, 2 out]
          }
          frame "Relay", "Solenoid" {
            w225 = FALSE ("Visible")
            n120 = property on="Motor" class="Clust (strict)"("Visible"=w225) -> ()  [unwired: 2 in, 2 out]
            n121 = property on="Test Slider" class="Slide (strict)"("Visible"=w225) -> ()  [unwired: 2 in, 2 out]
            n122 = Search and Replace String(input string=w226, search string="/Value  **", replace string="/Direction") -> (result string=w232:string)  [unwired: 5 in, 3 out]
            n123 = property on="Test Ring" class="Ring (strict)"("Visible"=w225) -> ()  [unwired: 2 in, 2 out]
            n124 = call <vilib>:"NT Read String.vi"("Name"=w232) -> ("String"=w230:string)  [unwired: 9 in, 1 out]
            n125 = Equal?(x="Both directions", y=w230) -> (x = y?=w228:bool)
            n126 = Not(x=w228) -> (.not. x?=w229:bool)
            n127 = property on="Rev/Fwd" class="Clust (strict)"("Visible"=w228) -> ()  [unwired: 2 in, 2 out]
            n128 = property on="On/Off" class="Bool (strict)"("Visible"=w229, "Caption.Text"=w227) -> ()  [unwired: 2 in, 2 out]
          }
          frame "Compressor", "Digital Out" {
            w235 = FALSE ("Visible")
            # "Get direction and finish"
            n129 = property on="Motor" class="Clust (strict)"("Visible"=w235) -> ()  [unwired: 2 in, 2 out]
            n130 = property on="Test Slider" class="Slide (strict)"("Visible"=w235) -> ()  [unwired: 2 in, 2 out]
            n131 = property on="Test Ring" class="Ring (strict)"("Visible"=w235) -> ()  [unwired: 2 in, 2 out]
            n132 = property on="On/Off" class="Bool (strict)"("Visible"=TRUE, "Caption.Text"=w236) -> ()  [unwired: 2 in, 2 out]
            n133 = property on="Rev/Fwd" class="Clust (strict)"("Visible"=FALSE) -> ()  [unwired: 2 in, 2 out]
          }
          frame "Camera" {
            n134 = call <vilib>:"Get Last Path Segment.vi"("String in"=w243) -> ("String out"=w244:string)  [unwired: 10 in]
            n135 = property on="On/Off" class="Bool (strict)"("Visible"=FALSE) -> ()  [unwired: 2 in, 2 out]
            n136 = property on="Motor" class="Clust (strict)"("Visible"=FALSE) -> ()  [unwired: 2 in, 2 out]
            n137 = property on="Rev/Fwd" class="Clust (strict)"("Visible"=FALSE) -> ()  [unwired: 2 in, 2 out]
            n138 = case shown="\"White Balance  **\"" w244 {
              tunnel: w243 -> [w250 w259 w268 w277 w286 _ w292]
              tunnel: w242 -> [w248 w256 w265 w274 w283 _ _]
              frame "Size  **" {
                n139 = Index Array(array=w248) -> (element=w247:cluster{string[]})  [unwired: 1 in]
                n140 = call <vilib>:"NT Read String.vi"("Name"=w250) -> ("String"=w249:string)  [unwired: 9 in, 1 out]
                n141 = Unbundle(w247) -> (w245:string[])
                n142 = Match First String(2:w245, 3:w249) -> (0:w246:i32)  [unwired: 1 out]
                n143 = property on="Test Ring" class="Ring (strict)"("Value"=w246, "Strings []"=w245) -> ()  [unwired: 2 in, 2 out]
                n144 = property on="Test Ring" class="Ring (strict)"("Visible"=TRUE) -> ()  [unwired: 2 in, 2 out]
                n145 = property on="Test Slider" class="Slide (strict)"("Visible"=FALSE) -> ()  [unwired: 2 in, 2 out]
              }
              frame "White Balance  **" {
                n146 = Index Array(array=w256, index=1) -> (element=w257:cluster{string[]})
                n147 = call <vilib>:"NT Read String.vi"("Name"=w259) -> ("String"=w258:string)  [unwired: 9 in, 1 out]
                n148 = Unbundle(w257) -> (w254:string[])
                n149 = Match First String(2:w254, 3:w258) -> (0:w253:i32)  [unwired: 1 out]
                n150 = property on="Test Ring" class="Ring (strict)"("Value"=w253, "Strings []"=w254) -> ()  [unwired: 2 in, 2 out]
                n151 = property on="Test Ring" class="Ring (strict)"("Visible"=TRUE) -> ()  [unwired: 2 in, 2 out]
                n152 = property on="Test Slider" class="Slide (strict)"("Visible"=FALSE) -> ()  [unwired: 2 in, 2 out]
              }
              frame "Exposure  **" {
                n153 = Index Array(array=w265, index=2) -> (element=w266:cluster{string[]})
                n154 = call <vilib>:"NT Read String.vi"("Name"=w268) -> ("String"=w267:string)  [unwired: 9 in, 1 out]
                n155 = Unbundle(w266) -> (w262:string[])
                n156 = Match First String(2:w262, 3:w267) -> (0:w263:i32)  [unwired: 1 out]
                n157 = property on="Test Ring" class="Ring (strict)"("Value"=w263, "Strings []"=w262) -> ()  [unwired: 2 in, 2 out]
                n158 = property on="Test Ring" class="Ring (strict)"("Visible"=TRUE) -> ()  [unwired: 2 in, 2 out]
                n159 = property on="Test Slider" class="Slide (strict)"("Visible"=FALSE) -> ()  [unwired: 2 in, 2 out]
              }
              frame "Exposure Priority  **" {
                n160 = Index Array(array=w274, index=3) -> (element=w275:cluster{string[]})
                n161 = call <vilib>:"NT Read String.vi"("Name"=w277) -> ("String"=w276:string)  [unwired: 9 in, 1 out]
                n162 = Unbundle(w275) -> (w271:string[])
                n163 = Match First String(2:w271, 3:w276) -> (0:w272:i32)  [unwired: 1 out]
                n164 = property on="Test Ring" class="Ring (strict)"("Value"=w272, "Strings []"=w271) -> ()  [unwired: 2 in, 2 out]
                n165 = property on="Test Ring" class="Ring (strict)"("Visible"=TRUE) -> ()  [unwired: 2 in, 2 out]
                n166 = property on="Test Slider" class="Slide (strict)"("Visible"=FALSE) -> ()  [unwired: 2 in, 2 out]
              }
              frame "Color Enable  **" {
                n167 = Index Array(array=w283, index=4) -> (element=w284:cluster{string[]})
                n168 = call <vilib>:"NT Read String.vi"("Name"=w286) -> ("String"=w285:string)  [unwired: 9 in, 1 out]
                n169 = Unbundle(w284) -> (w280:string[])
                n170 = Match First String(2:w280, 3:w285) -> (0:w281:i32)  [unwired: 1 out]
                n171 = property on="Test Ring" class="Ring (strict)"("Value"=w281, "Strings []"=w280) -> ()  [unwired: 2 in, 2 out]
                n172 = property on="Test Ring" class="Ring (strict)"("Visible"=TRUE) -> ()  [unwired: 2 in, 2 out]
                n173 = property on="Test Slider" class="Slide (strict)"("Visible"=FALSE) -> ()  [unwired: 2 in, 2 out]
              }
              frame Default {
                n174 = property on="Test Ring" class="Ring (strict)"("Visible"=FALSE) -> ()  [unwired: 2 in, 2 out]
                n175 = property on="Test Slider" class="Slide (strict)"("Visible"=FALSE) -> ()  [unwired: 2 in, 2 out]
              }
              frame "Brightness  **", "Color Level  **", "Compression  **", "FPS  **", "Sharpness  **" {
                n176 = call <vilib>:"NT Read Number.vi"("Name"=w292) -> ("Numeric"=w291:dbl)  [unwired: 9 in, 1 out]
                n177 = local write "Test Slider"(w291) -> ()
                n178 = property on="Test Slider" class="Slide (strict)"("Visible"=TRUE, "Scale.Maximum"=100.0 ("Scale.Range:Maximum")) -> ()  [unwired: 2 in, 2 out]
                n179 = property on="Test Ring" class="Ring (strict)"("Visible"=FALSE) -> ()  [unwired: 2 in, 2 out]
              }
            }
          }
        }
        n180 = property on="Progress" class="Clust (strict)"("Visible"=FALSE) -> ()  [unwired: 2 in, 2 out]
      }
      event "Test Name": Mouse Enter {
        # "Populate the ring with the list of tests"
        n181 = event-data() -> ()  [unwired: 1 in, 1 out]
        n182 = call <vilib>:"NT Read String Array.vi"("Name"="/TestMode/TestList") -> ("String Array"=w301:string[])  [unwired: 9 in, 1 out]
        n183 = Build Array (concatenate)("Select the test to run...", w301) -> (w300:string[])
        n184 = property on="Test Name" class="Ring (strict)"("Strings []"=w300) -> ()  [unwired: 2 in, 2 out]
      }
      event "Test Name": Value Change {
        w304 = FALSE ("Visible")
        # "Tell the robot the test name to run"
        n185 = event-data() -> ("NewVal"=w308:u16)  [unwired: 1 in]
        n186 = property on="Test Name" class="Ring (strict)"() -> ("Strings []"=w309:string[])  [unwired: 2 in, 2 out]
        n187 = local write "Progress"(T8 {"Test Progress"=0, "Test Progress Text"=""} ("Progress")) -> ()
        n188 = Index Array(array=w309, index=w308) -> (element=w307:string)
        n189 = call <vilib>:"NT Write String.vi"("String"=w307, "Name"="/TestMode/TestName") -> ()  [unwired: 9 in, 1 out]
        n190 = property on="Progress" class="Clust (strict)"("Visible"=TRUE) -> ()  [unwired: 2 in, 2 out]
        n191 = property on="Motor" class="Clust (strict)"("Visible"=w304) -> ()  [unwired: 2 in, 2 out]
        n192 = property on="Test Slider" class="Slide (strict)"("Visible"=w304) -> ()  [unwired: 2 in, 2 out]
        n193 = property on="On/Off" class="Bool (strict)"("Visible"=w304) -> ()  [unwired: 2 in, 2 out]
        n194 = property on="Rev/Fwd" class="Clust (strict)"("Visible"=w304) -> ()  [unwired: 2 in, 2 out]
        n195 = property on="Test Ring" class="Ring (strict)"("Visible"=w304) -> ()  [unwired: 2 in, 2 out]
      }
      event "Select Auto": Mouse Enter {
        # "Populate the combo box with the list of autonomous options"
        n196 = event-data() -> ()  [unwired: 1 in, 1 out]
        n197 = call <vilib>:"NT Read String Array.vi"("Name"="Auto List") -> ("String Array"=w311:string[])  [unwired: 9 in, 1 out]
        n198 = property on="Select Auto" class="CmbBox"("Strings[]"=w311) -> ()  [unwired: 2 in, 2 out]
      }
      event "Select Auto": Value Change {
        # "User modified the Auto Selection. Write to NT variable so robot knows."
        n199 = event-data() -> ("NewVal"=w315:string)  [unwired: 1 in]
        n200 = call <vilib>:"NT Write String.vi"("String"=w315, "Name"="Auto Selector") -> ()  [unwired: 9 in, 1 out]
      }
      event "Command Selection": Value Change {
        # "Get the params and show in table"
        n201 = event-data() -> ("NewVal"=w322:i32)  [unwired: 1 in]
        n202 = property on="Command Selection" class="MCListbox (strict)"() -> ("ItemNames"=w320:string[][])  [unwired: 2 in, 2 out]
        n203 = call <vilib>:"WPI_DashboardUpdate Command Params.vi"("NewVal"=w322, "Commands"=w320, "Param Tbl"=w321) -> ()  [unwired: 8 in, 1 out]
      }
      event "Execute Command": Value Change {
        # "Started one, Unique ID holds\nresponse"
        n204 = event-data() -> ()  [unwired: 1 in, 1 out]
        n205 = property on="Command Selection" class="MCListbox (strict)"() -> ("ItemNames"=w334:string[][])  [unwired: 2 in, 2 out]
        n206 = Index Array(array=w334, index (row)="Command Selection", index (col)=0) -> (element=w332:string)
        n207 = call <vilib>:"Invoke Commands.vi"("Command Params"="Command Params", "Function Name"=w332) -> ("Params"=w328:u8, "Started"=w327:bool)  [unwired: 7 in, 1 out]
        n208 = Array Subset(array="Command Params", length (row)=w328) -> (w329:string[][])  [unwired: 3 in]
        n209 = Select(t="Executing" ("Cmd Status"), s=w327, f="" ("Cmd Status")) -> (s? t:f=→"Cmd Status":string)
      }
      event "Command Selection": Double Click {
        n210 = event-data() -> ("Row"=w344:i32)  [unwired: 1 in]
        n211 = property on="Command Selection" class="MCListbox (strict)"() -> ("ItemNames"=w347:string[][])  [unwired: 2 in, 2 out]
        n212 = local read "Command Params"() -> (w342:string[][])
        n213 = Index Array(array=w347, index (row)=w344, index (col)=0) -> (element=w345:string)
        n214 = call <vilib>:"Invoke Commands.vi"("Command Params"=w342, "Function Name"=w345) -> ("Params"=w341:u8, "Started"=w336:bool)  [unwired: 7 in, 1 out]
        n215 = Array Subset(array=w342, length (row)=w341) -> (w340:string[][])  [unwired: 3 in]
        n216 = Select(t="Executing" ("Cmd Status"), s=w336, f="" ("Cmd Status")) -> (s? t:f=w337:string)
        n217 = local write "Cmd Status"(w337) -> ()
      }
      event "CheckList": Double Click {
        # "Shift clears all"
        # "Update symbols on the listbox"
        n218 = event-data() -> ("PlatMods.Shift"=w350:bool, "Row"=w352:i32)  [unwired: 1 in]
        n219 = case shown="True" w350 {
          tunnel: w352 -> [w356 _]
          tunnel: 1 -> [w355 _]
          frame False {
            n220 = property on="CheckList" class="LstBox (strict)"() -> ("Item Symbols"=w354:i32[])  [unwired: 2 in, 2 out]
            n221 = Replace Array Subset(array=w354, new element=w355, index=w356) -> (w353:i32[])
            n222 = property on="CheckList" class="LstBox (strict)"("Item Symbols"=w353) -> ()  [unwired: 2 in, 2 out]
          }
          frame True {
            w357 = 0 ("Top Row")
            n223 = property on="CheckList" class="LstBox (strict)"() -> ("Number of Rows"=w359:u32)  [unwired: 2 in, 2 out]
            n224 = Initialize Array(0, w359) -> (w358:i32[])
            n225 = property on="CheckList" class="LstBox (strict)"("Top Row"=w357, "Value"=w357, "Item Symbols"=w358) -> ()  [unwired: 2 in, 2 out]
          }
        }
      }
      event "CheckList": Key Down {
        # "Update symbols on the listbox\nLeft and right keys check and uncheck"
        n226 = event-data() -> ("VKey"=w364:T22)  [unwired: 1 in]
        n227 = case shown="\"Left\", \"Right\"" w364 {
          selector: w364 -> [w369 _]
          tunnel: eventvkey."Left" ("VKey") -> [w367 _]
          frame "Left", "Right" {
            n228 = Equal?(x=w367, y=w369) -> (x = y?=w368:bool)
            n229 = Select(t=0, s=w368, f=1) -> (s? t:f=w370:i32)
            n230 = property on="CheckList" class="LstBox (strict)"() -> ("Item Symbols"=w373:i32[])  [unwired: 2 in, 2 out]
            n231 = Replace Array Subset(array=w373, new element=w370, index="CheckList") -> (w372:i32[])
            n232 = property on="CheckList" class="LstBox (strict)"("Item Symbols"=w372) -> ()  [unwired: 2 in, 2 out]
          }
          frame Default {
          }
        }
      }
      event "DB Camera Config": Value Change {
        # "Show or hide the cluster of controls, store in ini file"
        n233 = event-data() -> ("NewVal"=w378:bool)  [unwired: 1 in]
        n234 = case shown="False" w378 {
          tunnel: w377 -> [w387 _]
          tunnel: [w380 w398] -> w376
          tunnel: w375 -> [w379 w398]
          frame False {
            w394 = "Camera"
            w397 = FALSE ("Visible")
            n235 = local read "Camera Settings"() -> (w386:T3)
            n236 = Index Array(array=w387) -> (element=w390:cluster{string[]})  [unwired: 1 in]
            n237 = Unbundle(w386) -> ("Frame Rate"=w385:i32, "Compression"=w384:i32, "Size"=w388:u16)
            n238 = Unbundle(w390) -> (w389:string[])
            n239 = Index Array(array=w389, index=w388) -> (element=w383:string)
            n240 = call-poly <vilib>:"Write Key.vi"("section"=w394, "value"=w383, "key"="Size", "refnum"=w379) -> ("refnum out"=w396:T20)  [unwired: 2 in, 5 out]
            n241 = call-poly <vilib>:"Write Key.vi"("section"=w394, "value"=w385, "key"="FrameRate", "refnum"=w396) -> ("refnum out"=w395:T20)  [unwired: 1 in, 6 out]
            n242 = property on="Camera Settings" class="Clust (strict)"("Visible"=w397) -> ()  [unwired: 2 in, 2 out]
            n243 = local write "DB Camera Config"(w397) -> ()
            n244 = call-poly <vilib>:"Write Key.vi"("section"=w394, "value"=w384, "key"="Compression", "refnum"=w395) -> ("refnum out"=w381:T20)  [unwired: 1 in, 6 out]
            n245 = call <vilib>:"Close Config Data.vi"("refnum"=w381) -> ("file path"=w382:path)  [unwired: 2 in, 8 out]
            n246 = call <vilib>:"Open Config Data.vi"("configuration file path"=w382) -> ("refnum"=w380:T20)  [unwired: 8 in, 2 out]
          }
          frame True {
            n247 = property on="Camera Settings" class="Clust (strict)"("Visible"=TRUE) -> ()  [unwired: 2 in, 2 out]
          }
        }
      }
      event "Camera Settings": Value Change {
        # "Update summary string when any elements of DB camera change"
        n248 = event-data() -> ("NewVal"=w412:T3)  [unwired: 1 in]
        n249 = Index Array(array=w408) -> (element=w407:cluster{string[]})  [unwired: 1 in]
        n250 = Unbundle(w412) -> ("Frame Rate"=w403:i32, "Compression"=w402:i32, "Size"=w405:u16)
        n251 = Unbundle(w407) -> (w406:string[])
        n252 = Index Array(array=w406, index=w405) -> (element=w404:string)
        n253 = Format Into String(format string="%s   %dfps   %d%%", w404, w403, w402) -> (resulting string=w409:string)  [unwired: 2 in, 1 out]
        n254 = Build Array(w409) -> (w410:string[])
        n255 = property on="DB Camera Config" class="Bool (strict)"("Strings [4]"=w410) -> ()  [unwired: 2 in, 2 out]
      }
      event "Motor.Enable": Value Change {
        # "When the test mode otor enable helper is set, update that\ntree row item's value"
        n256 = event-data() -> ("NewVal"=w419:bool)  [unwired: 1 in]
        n257 = Unbundle("Motor") -> ("Value"=w418:dbl)  [unwired: 1 out]
        n258 = Select(t=w418, s=w419, f=0.0) -> (s? t:f=w416:dbl)
        n259 = call <vilib>:"NT Write Number.vi"("Numeric"=w416, "Name"=w415) -> ()  [unwired: 9 in, 1 out]
      }
      event "Test Slider": Value Change {
        # "When the test mode slider helper is set, update that\ntree row item's value"
        n260 = event-data() -> ("NewVal"=w423:dbl)  [unwired: 1 in]
        n261 = call <vilib>:"NT Write Number.vi"("Numeric"=w423, "Name"=w424) -> ()  [unwired: 9 in, 1 out]
      }
      event "On/Off": Value Change {
        # "When the test mode on/off helper value is set, update that\ntree row item's value"
        n262 = event-data() -> ("NewVal"=w429:bool)  [unwired: 1 in]
        n263 = Boolean To (0,1)(Boolean=w429) -> (0, 1=w428:i16)
        n264 = call <vilib>:"NT Write Number.vi"("Numeric"=w428, "Name"=w427) -> ()  [unwired: 9 in, 1 out]
      }
      event "Rev/Fwd": Value Change {
        # "When the test mode helper value for relays is set, update that\ntree row item's value"
        n265 = event-data() -> ("NewVal.Forward"=w438:bool, "NewVal.Reverse"=w437:bool)  [unwired: 1 in]
        n266 = Boolean To (0,1)(Boolean=w438) -> (0, 1=w434:i16)
        n267 = Boolean To (0,1)(Boolean=w437) -> (0, 1=w436:i16)
        n268 = Negate(x=w436) -> (-x=w435:i16)
        n269 = Add(x=w434, y=w435) -> (x+y=w433:i16)
        n270 = call <vilib>:"NT Write Number.vi"("Numeric"=w433, "Name"=w432) -> ()  [unwired: 9 in, 1 out]
      }
      event "Test Ring": Value Change {
        # "When a test mode helper value is selected from the ring,\nset the tree item's variable to the string value"
        n271 = event-data() -> ("NewVal"=w443:u16)  [unwired: 1 in]
        n272 = property on="Test Ring" class="Ring (strict)"() -> ("Strings []"=w444:string[])  [unwired: 2 in, 2 out]
        n273 = Index Array(array=w444, index=w443) -> (element=w442:string)
        n274 = call <vilib>:"NT Write String.vi"("String"=w442, "Name"=w441) -> ()  [unwired: 9 in, 1 out]
      }
      event "Rec Mode": Value Change {
        # "Update globals for recording mode and path to read log from.\nClear when logging and let NetworkTables set path for vision to\nuse."
        n275 = event-data() -> ("NewVal"=w456:enum32{"Stop", "Record", "Playback"})  [unwired: 1 in]
        n276 = global write "WPI_DashboardLogging Global.vi" "Logging Filename"(path "") -> ()
        n277 = global write "WPI_DashboardLogging Global.vi" "Recording"(w456) -> ()
        n278 = case shown="\"Playback\"" w456 {
          tunnel: w455 -> [_ w458 w467]
          tunnel: [_ _ w466] -> w452
          tunnel: [_ _ w465] -> _
          tunnel: w450 -> [_ _ w463]
          tunnel: cluster{i32, i32} {-250, 170} -> [_ _ w462]
          tunnel: [_ _ T23 {"Image Size"=TRUE, "Image Type"=TRUE, "Pixel Value"=TRUE, "ROI Information"=TRUE, "Zoom Factor"=FALSE} ("Image Information Shown:All Elements")] -> w448
          tunnel: [_ _ TRUE ("Zoom Factor")] -> w447
          tunnel: w446 -> [_ _ w459]
          frame Default {
          }
          frame "Stop", "Record" {
            # "Place Window too"
            n279 = invoke class="VI" method="FP.Close"(reference=w458) -> (reference out=w457:refnum<vi>)  [unwired: 2 in, 2 out]
            n280 = invoke class="VI" method="Abort VI"(reference=w457) -> ()  [unwired: 2 in, 3 out]
          }
          frame "Playback" {
            n281 = call "Open Playback Panel.vi"("Offset"=w462, "DB VI Ref"=w463, "Playback in"=w467) -> ("Playback out"=w464:refnum<vi>)  [unwired: 8 in]
            n282 = register-events(w464, w459) -> (reference out=w466:refnum<event-registration>, error out=w465:errorcluster)  [unwired: 2 in]
          }
        }
        n283 = property on="Camera Image" class="ImageControl"("Image Information Shown"=w448, "Image Information Visible"=w447) -> ()  [unwired: 2 in, 2 out]
        n284 = call <vilib>:"WPI_DashboardNT Log FieldName Cache.vi"("Operation"=enum16{"Lookup/Add", "Index", "Clear"}."Clear") -> ()  [unwired: 8 in, 3 out]
      }
      event Panel Close {
        w469 = enum32{"Stop", "Record", "Playback"}."Stop" ("Rec Mode")
        # "Playback window has been closed, abort"
        n285 = event-data() -> ()  [unwired: 1 in, 4 out]
        n286 = local write "Rec Mode"(w469) -> ()
        n287 = global write "WPI_DashboardLogging Global.vi" "Recording"(w469) -> ()
      }
      event Panel Close {
        # "Abort playback window and ourself"
        n288 = event-data() -> ()  [unwired: 1 in, 4 out]
        n289 = invoke class="VI" method="FP.Close"(reference=w475) -> (reference out=w474:refnum<vi>)  [unwired: 2 in, 2 out]
        n290 = invoke class="VI" method="Abort VI"(reference=w474) -> (error out=w473:errorcluster)  [unwired: 2 in, 2 out]
        n291 = invoke class="VI" method="Abort VI"(error in=w473) -> ()  [unwired: 2 in, 3 out]
      }
      event User Event {
        n292 = event-data() -> ("IDs"=w483:cluster{"RPC field ID":u16, "Unique ID":u16}, "String"=w482:string)  [unwired: 1 in]
        n293 = Bundle("IDs"=w483, "String"=w482) -> (w481:T10)  [unwired: 1 in]
        n294 = call <vilib>:"Retrieve RPC Response.vi"("RPC Response"=w481) -> ("Output"=w478:string[][])  [unwired: 10 in]
        n295 = Build Array (concatenate)(w476, w478) -> (w477:string[][])
        n296 = local write "Command Params"(w477) -> ()
        n297 = local write "Cmd Status"("" ("Cmd Status")) -> ()
      }
      event "Vision": Value Change {
        # "Enable/Disable Compression slider.\nHW USB is hard-coded into the camera"
        n298 = event-data() -> ("NewVal"=w490:u16)  [unwired: 1 in]
        n299 = Equal?(x=w490, y=u32 2 ("milliseconds to wait")) -> (x = y?=w488:bool)
        n300 = Select(t=T24."Disabled and Grayed Out" ("Disabled"), s=w488, f=T24."Enabled" ("Disabled")) -> (s? t:f=w485:T24)
        n301 = property on="Compression" class="Slide (strict)"("DisabledEnum"=w485) -> ()  [unwired: 2 in, 2 out]
      }
      event "Tree": Double Click {
        n302 = event-data() -> ("PlatMods"=w495:T27, "Tag"=w494:string)  [unwired: 1 in]
        n303 = Unbundle(w495) -> ("Shift"=w493:bool)  [unwired: 4 out]
        n304 = Not(x=w493) -> (.not. x?=w492:bool)
        n305 = call <vilib>:"NT Update Persistence.vi"("Persistence"=w492, "Name"=w494) -> ()  [unwired: 9 in, 1 out]
      }
    }
  }
  n306 = while {
    tunnel: w50 -> [w499]
    i -> [w502]
    stop <- FALSE stop-if-true
    n307 = Wait (ms)(milliseconds to wait=u32 100) -> ()  [unwired: 1 out]
    n308 = case shown="\"Stop\", Default" "Rec Mode" {
      tunnel: w502 -> [_ _ w515]
      tunnel: [u32 2829099 ("Base Color") u32 11141120 ("Target Color") w506] -> w498
      frame "Stop", Default {
        # "Reset the color, extra updates don't cost much"
      }
      frame "Record" {
      }
      frame "Playback" {
        # "Playback"
        n309 = Quotient & Remainder(x=w515, y=u32 50 ("milliseconds to wait")) -> (x-y*floor(x/y)=w512:u32)  [unwired: 1 out]
        n310 = Divide(x=w512, y=u32 50 ("milliseconds to wait")) -> (x/y=w509:dbl)
        n311 = Multiply(x=6.283185307179586, y=w509) -> (x*y=w513:dbl)
        n312 = Sine(x=w513) -> ()  [unwired: 1 out]
        n313 = call "Interpolate RGB Color.vi"("Target Color"=u32 30976, "Base Color"=u32 2829099) -> ("Result Color"=w506:u32)  [unwired: 9 in]
      }
    }
    n314 = property class="Pane"(reference=w499, "PaneColor"=w498) -> ()  [unwired: 1 in, 2 out]
  }
  n315 = local write "Dashboard Tab"(T2."Drive" ("Dashboard Tab")) -> ()
  n316 = property on="On/Off" class="Bool (strict)"("Visible"=w18) -> ()  [unwired: 2 in, 2 out]
  n317 = property on="Motor" class="Clust (strict)"("Visible"=w18) -> ()  [unwired: 2 in, 2 out]
  n318 = property on="Progress" class="Clust (strict)"("Visible"=w18) -> ()  [unwired: 2 in, 2 out]
  n319 = property on="Test Ring" class="Ring (strict)"("Visible"=w18) -> ()  [unwired: 2 in, 2 out]
  n320 = property on="Rev/Fwd" class="Clust (strict)"("Visible"=w18) -> ()  [unwired: 2 in, 2 out]
  n321 = property on="Camera Settings" class="Clust (strict)"("Visible"=w18) -> ()  [unwired: 2 in, 2 out]
  n322 = local write "DB Camera Config"(w18) -> ()
  n323 = local write "Command Params"(string[][] [] ("Command Params")) -> ()
  n324 = global write "WPI_DashboardLogging Global.vi" "Recording"(w44) -> ()
  n325 = local write "Rec Mode"(w44) -> ()
  n326 = while {
    tunnel: u16 1741 ("timeout ms (25000)") -> [w517]
    stop <- FALSE stop-if-true
    n327 = TCP Create Listener(10:w517) -> (0:w516:errorcluster, 3:w518:refnum<k5>)  [unwired: 4 in, 1 out]
    n328 = case shown="No Error" w516 {
      selector: w516 -> [w520 _]
      tunnel: w518 -> [w521 _]
      frame No Error {
        n329 = while {
          tunnel: w521 -> [w524]
          tunnel: w520 -> [w523]
          stop <- FALSE stop-if-true
          n330 = TCP Wait On Listener(8:w523, 11:w524) -> (0:w525:errorcluster, 4:w526:refnum<k5>)  [unwired: 2 in, 3 out]
          n331 = local write "TCP"(w526) -> ()
          n332 = case shown="No Error" w525 {
            frame No Error {
            }
            frame Error {
              n333 = Wait (ms)(milliseconds to wait=u32 1000) -> ()  [unwired: 1 out]
            }
          }
        }
      }
      frame Error {
        n334 = Wait (ms)(milliseconds to wait=u32 1000) -> ()  [unwired: 1 out]
      }
    }
  }
  n335 = local write "Command Selection"(u16 0 ("milliseconds to wait")) -> ()
  n336 = call "IMAQ Create"("Image Name"="Dashboard Image 2", "Image Type"=w2) -> ("New Image"=w1:T1)  [unwired: 2 in, 2 out]
  n337 = while {
    tunnel: w62 -> [w538]
    tunnel: w61 -> [_]
    tunnel: [w539] -> _
    tunnel: w1 -> [w529]
    i -> [w539]
    stop <- FALSE stop-if-true
    # "Optionally read the DB image,\nlog, or retrieve images from a\nlogged match"
    n338 = local read "Rec Mode"() -> (w533:enum32{"Stop", "Record", "Playback"})
    n339 = local read "Camera IP"() -> (w531:string)
    n340 = call <vilib>:"WPI_CameraRead MJPG for Dashboard.vi"("Camera Settings"="Camera Settings", "Rec Mode"=w533, "Camera IP"=w531, "Camera Mode"="Vision", "Refnum in"=w538) -> ("Active"=w536:bool, "Refnum out"=w537:T1, "FPS"=w535:dbl, "Bandwidth (Mbps)"=w530:dbl)  [unwired: 3 in]
    "Mbps" <- w530
    n341 = case shown="True" w536 {
      tunnel: w537 -> [_ w554]
      tunnel: w530 -> [_ w553]
      tunnel: w535 -> [_ w552]
      tunnel: w529 -> [_ w545]
      frame False {
        w541 = u32 1985280 ("Color Box")
        # "Sleep for 500ms"
        n342 = Bundle("Color Box"=w541, "Color Box"=w541) -> (w543:cluster{"Color Box":u32, "Color Box":u32})  [unwired: 1 out]
        n343 = Build Array(w543) -> (w542:cluster{"Color Box":u32, "Color Box":u32}[])
        n344 = property on="Mbps LED" class="Bool (strict)"("Colors [4]"=w542) -> ()  [unwired: 2 in, 2 out]
        n345 = Wait Until Next ms Multiple(millisecond multiple=u32 500) -> ()  [unwired: 1 out]
      }
      frame True {
        # "Here is where you would annotate,\npossibly process, and display the image"
        # "Update Mbps LED"
        n346 = call "IMAQ Clear Overlay"("Image"=w554) -> ("error out"=w558:errorcluster, "Image Out"=w547:T1)  [unwired: 2 in, 7 out]
        n347 = case shown="Default" w553 {
          tunnel: [u32 6618880 ("Color Box") u32 16776722 ("Color Box") u32 16716800 ("Color Box")] -> w555
          frame Default {
          }
          frame 4, 5 {
          }
          frame 6.. {
          }
        }
        n348 = Unbundle By Name(w558) -> ("status"=w559:bool)
        n349 = Bundle("Color Box"=w555, "Color Box"=w555) -> (w557:cluster{"Color Box":u32, "Color Box":u32})  [unwired: 1 out]
        n350 = call-poly <vilib>:"NT Read Value.vi"("Name"="Flip") -> ("Boolean"=w550:bool)  [unwired: 9 in, 1 out]
        "Camera Reversed" <- w550
        n351 = property on="Image Message" class="Str"("Visible"=w559) -> ()  [unwired: 2 in, 2 out]
        n352 = Build Array(w557) -> (w556:cluster{"Color Box":u32, "Color Box":u32}[])
        n353 = property on="Mbps LED" class="Bool (strict)"("Colors [4]"=w556) -> ()  [unwired: 2 in, 2 out]
        n354 = call "IMAQ ImageToImage 2"("Image Dst"=w547, "Image Src (Small)"=w545, "Image Src (Large)"=w547) -> ("Image Dst Out"=w546:T1)  [unwired: 7 in, 1 out]
        n355 = case shown="True" w550 {
          tunnel: w546 -> [w560 w563]
          tunnel: [w560 w562] -> w549
          frame False {
          }
          frame True {
            n356 = call "IMAQ Rotate"("Angle (degrees)"=sgl 180.0, "Image Src"=w563) -> ("Image Dst Out"=w562:T1)  [unwired: 8 in, 1 out]
          }
        }
        n357 = call "Vision Assistant"("Image In"=w549) -> ("Image Out"=→"Camera Image":T1)  [unwired: 25 in, 1 out]
        "fps" <- w552
      }
    }
  }
  n358 = while {
    tunnel: [w576] -> _
    tunnel: w1 -> [w567]
    i -> [w576]
    stop <- FALSE stop-if-true
    # "Optionally read the DB image,\nlog, or retrieve images from a\nlogged match"
    n359 = local read "Rec Mode"() -> (w571:enum32{"Stop", "Record", "Playback"})
    n360 = local read "Camera IP"() -> (w569:string)
    n361 = call <vilib>:"WPI_CameraRead MJPG for Dashboard.vi"("Camera Settings"="Camera Settings 2", "Rec Mode"=w571, "Camera IP"=w569, "Camera Mode"="Vision 2", "Refnum in"=w567) -> ("Active"=w574:bool, "Refnum out"=w575:T1, "FPS"=w573:dbl, "Bandwidth (Mbps)"=w568:dbl)  [unwired: 3 in]
    "Mbps 2" <- w568
    n362 = case shown="True" w574 {
      tunnel: w575 -> [_ w585]
      tunnel: w568 -> [_ w584]
      tunnel: w573 -> [_ w583]
      frame False {
        w578 = u32 1985280 ("Color Box")
        # "Sleep for 500ms"
        n363 = Bundle("Color Box"=w578, "Color Box"=w578) -> (w580:cluster{"Color Box":u32, "Color Box":u32})  [unwired: 1 out]
        n364 = Build Array(w580) -> (w579:cluster{"Color Box":u32, "Color Box":u32}[])
        n365 = property on="Mbps LED" class="Bool (strict)"("Colors [4]"=w579) -> ()  [unwired: 2 in, 2 out]
        n366 = Wait Until Next ms Multiple(millisecond multiple=u32 500) -> ()  [unwired: 1 out]
      }
      frame True {
        # "Here is where you would annotate,\npossibly process, and display the image"
        # "Update Mbps LED"
        n367 = call "IMAQ Clear Overlay"("Image"=w585) -> ("error out"=w589:errorcluster, "Image Out"=→"Camera Image 2":T1)  [unwired: 2 in, 7 out]
        n368 = case shown="Default" w584 {
          tunnel: [u32 6618880 ("Color Box") u32 16776722 ("Color Box") u32 16716800 ("Color Box")] -> w586
          frame Default {
          }
          frame 4, 5 {
          }
          frame 6.. {
          }
        }
        n369 = Unbundle By Name(w589) -> ("status"=w590:bool)
        n370 = Bundle("Color Box"=w586, "Color Box"=w586) -> (w588:cluster{"Color Box":u32, "Color Box":u32})  [unwired: 1 out]
        n371 = property on="Image Message" class="Str"("Visible"=w590) -> ()  [unwired: 2 in, 2 out]
        n372 = Build Array(w588) -> (w587:cluster{"Color Box":u32, "Color Box":u32}[])
        n373 = property on="Mbps LED" class="Bool (strict)"("Colors [4]"=w587) -> ()  [unwired: 2 in, 2 out]
        "fps 2" <- w583
      }
    }
  }
